vi "Auto_gear.vi"(7 "autoGearRate":u32=10, 11 "Enum in":T1) -> (3 "Enum out":T1)   [LabVIEW 2016]
uses:
  Controls/currentState.ctl
  Robot Global Data.vi
panel:
  in  "PDP esquerda 3":i32=13
  in  "PDP esquerda 2":i32=15
  in  "PDP direita 3":i32=1
  in  "PDP direita 2":i32=2
  out "Direita":dbl(graph)
  out "Esquerda":dbl(graph)
  in  "PDP esquerda":i32=14
  in  "PDP direita":i32
  in  "timeout":dbl=400.0
  in  "thUp":dbl=5.0
  in  "thDown":dbl=30.0
  out "LOW":bool
  out "HIGH":bool
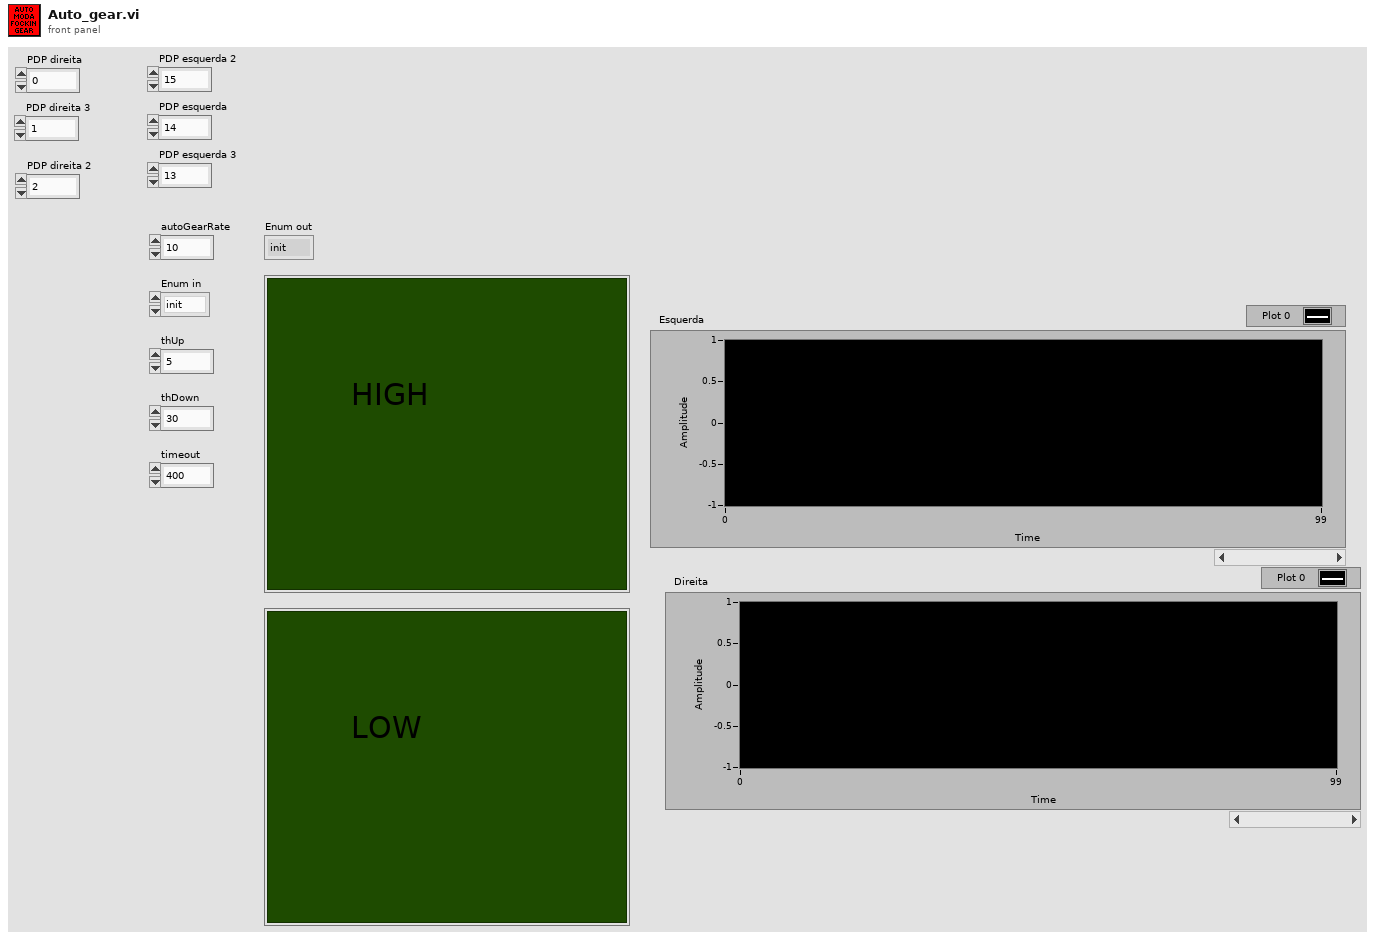
[diagram p1: front panel]
types:
  T1 = typedef "currentState.ctl" = enum16{"init", "gearUp", "gearDown"}
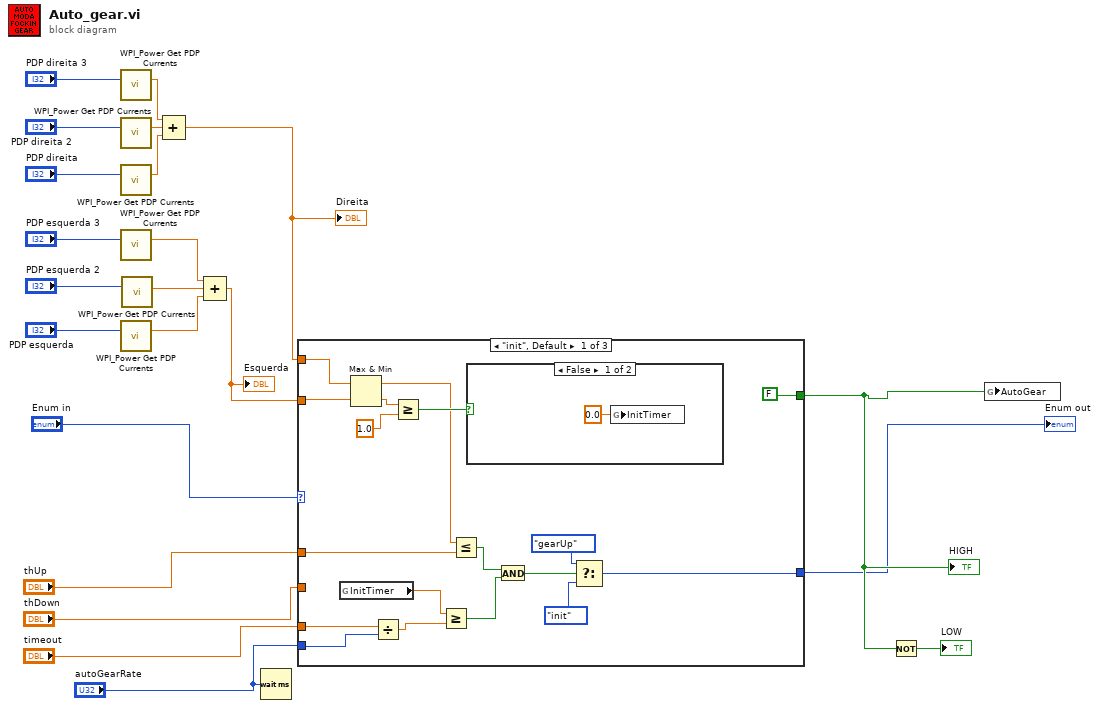
[diagram p0: block diagram]
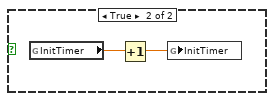
[diagram p2: hidden frame]
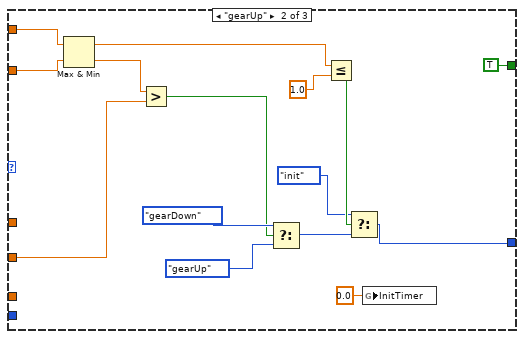
[diagram p3: hidden frame]
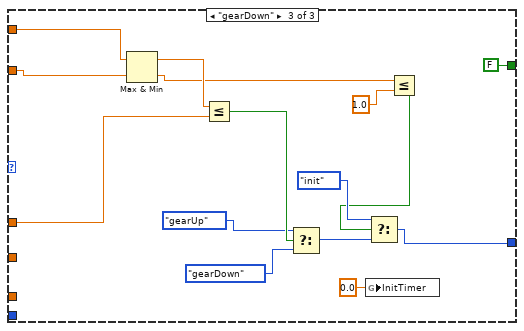
[diagram p4: hidden frame]
diagram:
  n1 = call <vilib>:"WPI_Power Get PDP Currents.vi"("PDP Channel"="PDP direita 3") -> ("current (A)"=w10:dbl)  [unwired: 12 in, 2 out]
  n2 = call <vilib>:"WPI_Power Get PDP Currents.vi"("PDP Channel"="PDP direita 2") -> ("current (A)"=w9:dbl)  [unwired: 12 in, 2 out]
  n3 = call <vilib>:"WPI_Power Get PDP Currents.vi"("PDP Channel"="PDP direita") -> ("current (A)"=w8:dbl)  [unwired: 12 in, 2 out]
  n4 = call <vilib>:"WPI_Power Get PDP Currents.vi"("PDP Channel"="PDP esquerda 3") -> ("current (A)"=w4:dbl)  [unwired: 12 in, 2 out]
  n5 = call <vilib>:"WPI_Power Get PDP Currents.vi"("PDP Channel"="PDP esquerda") -> ("current (A)"=w2:dbl)  [unwired: 12 in, 2 out]
  n6 = call <vilib>:"WPI_Power Get PDP Currents.vi"("PDP Channel"="PDP esquerda 2") -> ("current (A)"=w3:dbl)  [unwired: 12 in, 2 out]
  n7 = Compound Arithmetic op=ADD(w10, w9, w8) -> (w7:dbl)
  "Direita" <- w7
  n8 = Compound Arithmetic op=ADD(w4, w3, w2) -> (w1:dbl)
  "Esquerda" <- w1
  n9 = Wait (ms)(milliseconds to wait="autoGearRate") -> ()  [unwired: 1 out]
  n10 = case shown="\"init\", Default" "Enum in" {
    tunnel: [FALSE TRUE FALSE] -> w21
    tunnel: w7 -> [w39 w57 w66]
    tunnel: w1 -> [w38 w56 w65]
    tunnel: "timeout" -> [w35 _ _]
    tunnel: "autoGearRate" -> [w34 _ _]
    tunnel: "thUp" -> [w28 _ w62]
    tunnel: [w24 w51 w61] -> w17
    tunnel: "thDown" -> [_ w55 _]
    frame "init", Default {
      n11 = global read "Robot Global Data.vi" "InitTimer"() -> (w32:dbl)
      n12 = Max & Min(x=w39, y=w38) -> (max(x,y)=w23:dbl, min(x,y)=w29:dbl)
      n13 = Divide(x=w35, y=w34) -> (x/y=w33:dbl)
      n14 = Greater Or Equal?(x=w29, y=1.0) -> (x >= y?=w36:bool)
      n15 = Greater Or Equal?(x=w32, y=w33) -> (x >= y?=w31:bool)
      n16 = Less Or Equal?(x=w23, y=w28) -> (x <= y?=w30:bool)
      n17 = case shown="False" w36 {
        frame False {
          n18 = global write "Robot Global Data.vi" "InitTimer"(0.0 ("initTimer")) -> ()
        }
        frame True {
          n19 = global read "Robot Global Data.vi" "InitTimer"() -> (w42:dbl)
          n20 = Increment(x=w42) -> (x+1=w43:dbl)
          n21 = global write "Robot Global Data.vi" "InitTimer"(w43) -> ()
        }
      }
      n22 = And(x=w30, y=w31) -> (x .and. y?=w27:bool)
      n23 = Select(t=currentState."gearUp", s=w27, f=currentState."init") -> (s? t:f=w24:T1)
    }
    frame "gearUp" {
      n24 = Max & Min(x=w57, y=w56) -> (max(x,y)=w44:dbl, min(x,y)=w48:dbl)
      n25 = Greater?(x=w48, y=w55) -> (0:w52:bool)
      n26 = Select(t=currentState."gearDown", s=w52, f=currentState."gearUp") -> (s? t:f=w50:T1)
      n27 = Less Or Equal?(x=w44, y=1.0) -> (x <= y?=w47:bool)
      n28 = Select(t=currentState."init", s=w47, f=w50) -> (s? t:f=w51:T1)
      n29 = global write "Robot Global Data.vi" "InitTimer"(0.0 ("initTimer")) -> ()
    }
    frame "gearDown" {
      n30 = Max & Min(x=w66, y=w65) -> (max(x,y)=w64:dbl, min(x,y)=w63:dbl)
      n31 = Less Or Equal?(x=w64, y=w62) -> (x <= y?=w69:bool)
      n32 = Select(t=currentState."gearUp", s=w69, f=currentState."gearDown") -> (s? t:f=w70:T1)
      n33 = global write "Robot Global Data.vi" "InitTimer"(0.0 ("initTimer")) -> ()
      n34 = Less Or Equal?(x=w63, y=1.0) -> (x <= y?=w72:bool)
      n35 = Select(t=currentState."init", s=w72, f=w70) -> (s? t:f=w61:T1)
    }
  }
  "HIGH" <- w21
  "Enum out" <- w17
  n36 = Not(x=w21) -> (.not. x?=→"LOW":bool)
  n37 = global write "Robot Global Data.vi" "AutoGear"(w21) -> ()
